vi "needle.vi"(4 "center":cluster{"x":i32, "y":i32}={"x"=35, "y"=32}, 6 "size":i16=29, 7 "angle":dbl, 10 "pict in":picture) -> (3 "pict out":picture)   [LabVIEW 2011]
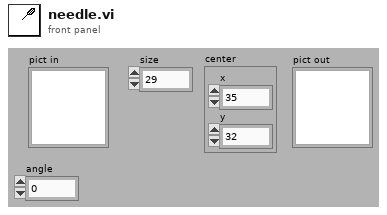
[diagram p1: front panel]
types:
  T1 = cluster{"Width":u16, "Style":enum32{"Solid", "Dash", "Dot", "DashDot", "DashDotDot"}}
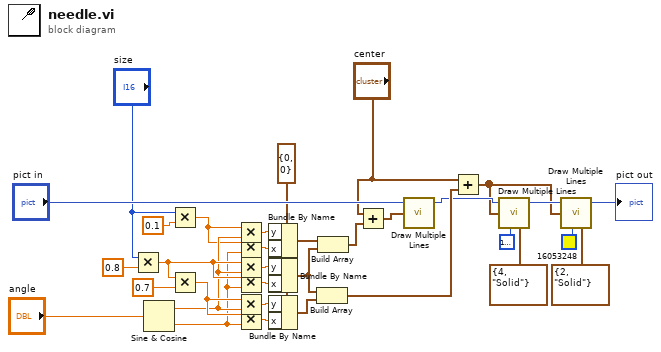
[diagram p0: block diagram]
diagram:
  w9 = cluster{"x":i16, "y":i16} {"x"=0, "y"=0}
  n1 = Multiply(x="size", y=0.8) -> (x*y=w26:dbl)
  n2 = Sine & Cosine(0:"angle") -> (1:w4:dbl, 2:w2:dbl)
  n3 = Multiply(x="size", y=0.1) -> (x*y=w1:dbl)
  n4 = Multiply(x=w26, y=0.7) -> (x*y=w24:dbl)
  n5 = Multiply(x=w1, y=w4) -> (x*y=w5:dbl)
  n6 = Multiply(x=w1, y=w2) -> (x*y=w3:dbl)
  n7 = Multiply(x=w26, y=w4) -> (x*y=w18:dbl)
  n8 = Multiply(x=w26, y=w2) -> (x*y=w19:dbl)
  n9 = Multiply(x=w24, y=w4) -> (x*y=w21:dbl)
  n10 = Multiply(x=w24, y=w2) -> (x*y=w22:dbl)
  n11 = Bundle By Name(cluster=w9, "y"=w5, "x"=w3) -> (w8:cluster{"x":i16, "y":i16})
  n12 = Bundle By Name(cluster=w9, "y"=w18, "x"=w19) -> (w31:cluster{"x":i16, "y":i16})
  n13 = Bundle By Name(cluster=w9, "y"=w21, "x"=w22) -> (w20:cluster{"x":i16, "y":i16})
  n14 = Build Array(w31, w20) -> (w17:cluster{"x":i16, "y":i16}[])
  n15 = Build Array(w8, w31) -> (w30:cluster{"x":i16, "y":i16}[])
  n16 = Add(x="center", y=w30) -> (x+y=w29:cluster{"x":i32, "y":i32}[])
  n17 = call <vilib>:"Draw Multiple Lines.vi"("picture"="pict in", "line endpoints"=w29) -> ("new picture"=w12:picture)  [unwired: 7 in]
  n18 = Add(x="center", y=w17) -> (x+y=w10:cluster{"x":i32, "y":i32}[])
  n19 = call <vilib>:"Draw Multiple Lines.vi"("picture"=w12, "line endpoints"=w10, "color(black)"=u32 16777222, "pen"=T1 {"Width"=4, "Style"=enum."Solid"}) -> ("new picture"=w11:picture)  [unwired: 5 in]
  n20 = call <vilib>:"Draw Multiple Lines.vi"("picture"=w11, "line endpoints"=w10, "color(black)"=u32 16053248, "pen"=T1 {"Width"=2, "Style"=enum."Solid"}) -> ("new picture"=→"pict out":picture)  [unwired: 5 in]
